vi "Write Attributes.vi"(7 "Name":string, 8 "error in":errorcluster, 9 "Reader":bool, 10 "Writer":bool, 11 "Proxy Status Msg in":refnum<class "Proxy Status Msg.lvclass">) -> (3 "Proxy Status Msg out":refnum<class "Proxy Status Msg.lvclass">)   [LabVIEW 2014, in "Proxy.lvlib" / "Proxy Status Msg.lvclass"]
uses:
  Proxy Status Msg.lvclass
  Proxy Status Msg.lvclass/Proxy Status Msg.ctl
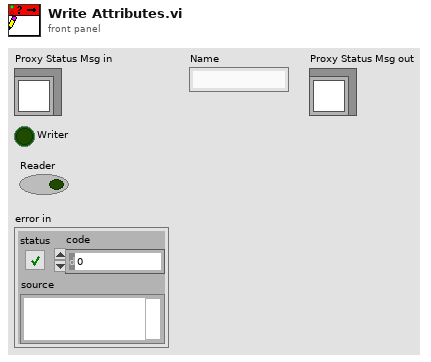
[diagram p1: front panel]
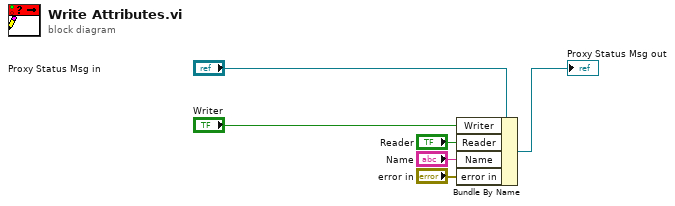
[diagram p0: block diagram]
diagram:
  n1 = Bundle By Name(cluster="Proxy Status Msg in", "Writer"="Writer", "Reader"="Reader", "Name"="Name", "error in"="error in") -> (→"Proxy Status Msg out":refnum<class "Proxy Status Msg.lvclass">)
